vi "Install Package.vi"(7 "Logger":refnum<class "Logger.lvclass">, 8 "error in (no error)":errorcluster, 11 "GitPackage in":refnum<class "GitPackage.lvclass">) -> (0 "error out":errorcluster, 3 "GitPackage out":refnum<class "GitPackage.lvclass">)   [LabVIEW 2020, in "GPack.lvlib" / "GitPackage.lvclass"]
uses:
  GitPackage.lvclass
  C:/dev/lv20CE/relink/lv-gpack/GPack/PackageAbstract/PackageAbstract.lvclass
  Logger/Logger.lvclass
  GitPackage.lvclass/GitPackage.ctl
  <vilib>/Hampel Software Engineering/Git API/Git API/GIT-api.lvclass/GIT-api.ctl
  <vilib>/Hampel Software Engineering/Git API/Git API/GIT-api.lvclass
  PackageAbstract/PackageAbstract.lvclass
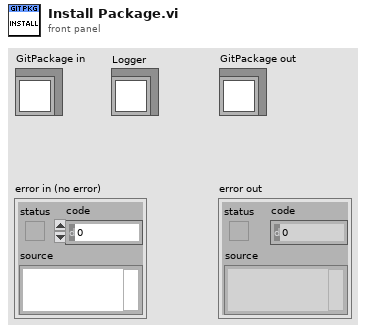
[diagram p1: front panel]
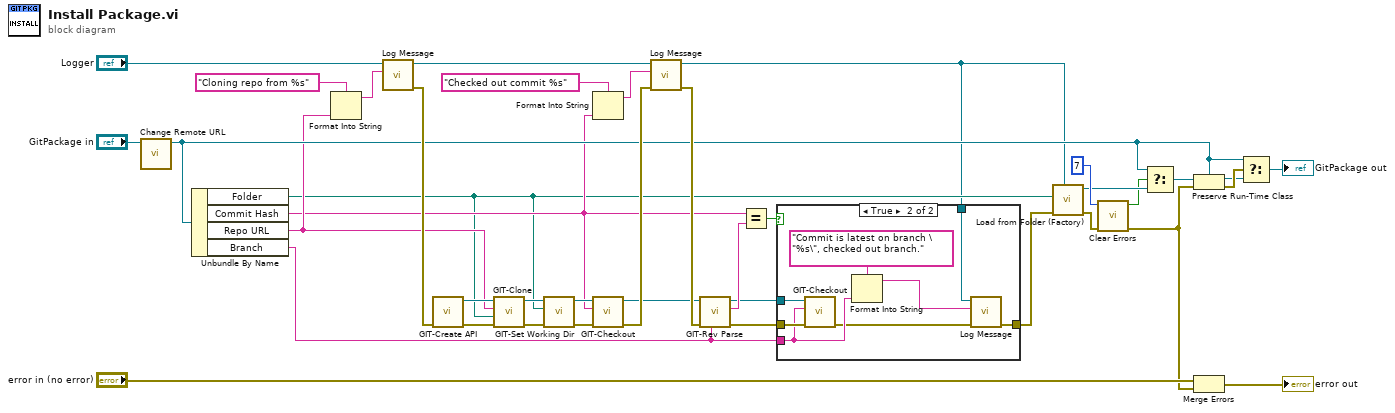
[diagram p0: block diagram]
diagram:
  n1 = call "Change Remote URL.vi"("GitPackage in"="GitPackage in") -> ("GitPackage out"=w19:refnum<class "GitPackage.lvclass">)  [unwired: 9 in, 1 out]
  n2 = Unbundle By Name(w19) -> ("Folder"=w7:path, "Commit Hash"=w9:string, "Repo URL"=w15:string, "Branch"=w3:string)
  n3 = Format Into String(format string="Cloning repo from %s", w15) -> (resulting string=w14:string)  [unwired: 2 in, 1 out]
  n4 = call "Log Message.vi"("Message"=w14, "Logger in"="Logger") -> ("error out"=w37:errorcluster, "Logger out"=w13:refnum<class "Logger.lvclass">)  [unwired: 8 in]
  n5 = call <vilib>:"GIT-Create API.vi"("error in"=w37) -> ("error out"=w35:errorcluster, "git-api out"=w33:refnum<class "GIT-api.lvclass">)  [unwired: 9 in]
  n6 = call <vilib>:"GIT-Clone.vi"("error in"=w35, "Local Path"=w7, "Repository URL"=w15, "git-api in"=w33) -> ("error out"=w31:errorcluster, "git-api out"=w28:refnum<class "GIT-api.lvclass">)  [unwired: 5 in, 1 out]
  n7 = call <vilib>:"GIT-Set Working Dir.vi"("error in"=w31, "Working Directory"=w7, "git-api in"=w28) -> ("error out"=w29:errorcluster, "git-api out"=w27:refnum<class "GIT-api.lvclass">)  [unwired: 7 in]
  n8 = Format Into String(format string="Checked out commit %s", w9) -> (resulting string=w11:string)  [unwired: 2 in, 1 out]
  n9 = call <vilib>:"GIT-Checkout.vi"("error in"=w29, "branch name"=w9, "git-api in"=w27) -> ("error out"=w38:errorcluster, "git-api out"=w10:refnum<class "GIT-api.lvclass">)  [unwired: 7 in]
  n10 = call "Log Message.vi"("error in (no error)"=w38, "Message"=w11, "Logger in"=w13) -> ("error out"=w39:errorcluster, "Logger out"=w2:refnum<class "Logger.lvclass">)  [unwired: 7 in]
  n11 = call <vilib>:"GIT-Rev Parse.vi"("param"=w3, "error in"=w39, "git-api in"=w10) -> ("error out"=w6:errorcluster, "std out"=w8:string, "git-api out"=w5:refnum<class "GIT-api.lvclass">)  [unwired: 6 in]
  n12 = Equal?(x=w9, y=w8) -> (x = y?=w4:bool)
  n13 = case shown="True" w4 {
    tunnel: w6 -> [w40 w48]
    tunnel: w5 -> [_ w47]
    tunnel: w3 -> [_ w46]
    tunnel: w2 -> [_ w44]
    tunnel: [w40 w41] -> w1
    frame False {
    }
    frame True {
      n14 = call <vilib>:"GIT-Checkout.vi"("error in"=w48, "branch name"=w46, "git-api in"=w47) -> ("error out"=w42:errorcluster)  [unwired: 7 in, 1 out]
      n15 = Format Into String(format string="Commit is latest on branch \"%s\", checked out branch.", w46) -> (resulting string=w43:string)  [unwired: 2 in, 1 out]
      n16 = call "Log Message.vi"("error in (no error)"=w42, "Message"=w43, "Logger in"=w44) -> ("error out"=w41:errorcluster)  [unwired: 7 in, 1 out]
    }
  }
  n17 = call "Load from Folder (Factory).vi"("Logger"=w2, "error in (no error)"=w1, "Folder"=w7) -> ("error out"=w26:errorcluster, "PackageAbstract out"=w24:refnum<class "PackageAbstract.lvclass">)  [unwired: 7 in]
  n18 = call <vilib>:"Clear Errors.vi"("error in (no error)"=w26, "specific error code to clear (0: all)"=7) -> ("error out"=w17:errorcluster, "specific error cleared?"=w23:bool)  [unwired: 4 in]
  n19 = Select(t=w19, s=w23, f=w24) -> (s? t:f=w22:refnum<class "PackageAbstract.lvclass">)
  n20 = Preserve Run-Time Class(object in=w22, error in=w17, 2:w19) -> (object out=w20:refnum<class "GitPackage.lvclass">, error out=w36:errorcluster)
  n21 = Merge Errors("error in (no error)", w17) -> (→"error out":errorcluster)
  n22 = Select(t=w19, s=w36, f=w20) -> (s? t:f=→"GitPackage out":refnum<class "GitPackage.lvclass">)
